vi "GA Send String.vi"(8 "error in (no error)":errorcluster caption="错误输入（无错误）", 9 "iOpenFlag":i32, 10 "iLen":i32, 11 "cString":string) -> (0 "error out":errorcluster caption="错误输出", 2 "function return":i32, 3 "cString out":string)   [LabVIEW 2015, in "GAS.lvlib"]
doc: "extern \"C\" __declspec(dllimport) int GA_SendString(char* cString,int iLen,int iOpenFlag=0);"
uses:
  <userlib>/BP_GAS/GAS.lvlib
  <userlib>/BP_GAS/GAS.dll
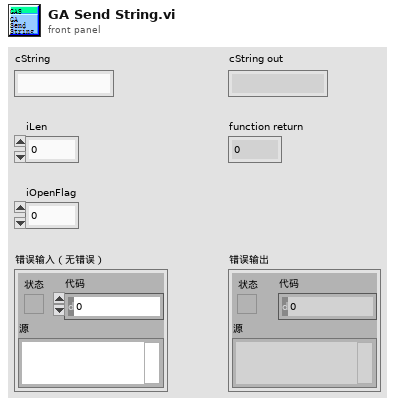
[diagram p1: front panel]
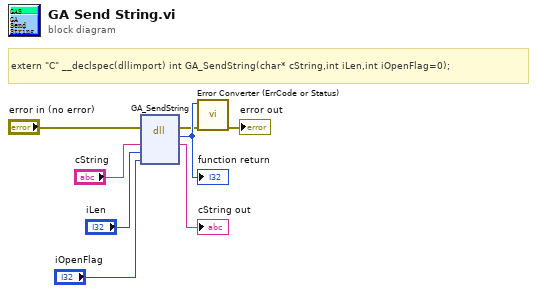
[diagram p0: block diagram]
diagram:
  # "extern \"C\" __declspec(dllimport) int GA_SendString(char* cString,int iLen,int iOpenFlag=0);"
  n1 = dll-call lib="E:/Program Files (x86)/National Instruments/LabVIEW 2015/user.lib/BP_GAS/GAS.*" fn="GA_SendString"(error in="error in (no error)", "cString"="cString", "iLen"="iLen", "iOpenFlag"="iOpenFlag") -> (error out=w2:errorcluster, w8:i32, "cString"=→"cString out":string)  [unwired: 4 in, 1 out]
  "function return" <- w8
  n2 = call "Error Converter (ErrCode or Status).vi"("error in (no error)"=w2, "error code"=w8) -> ("error out"=→"error out":errorcluster)  [unwired: 9 in]
